vi "UnittodB.vi"   [LabVIEW 2014]
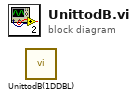
[diagram p0: block diagram]
diagram:
  n1 = call "UnittodB(1DDBL).vi"() -> ()  [unwired: 11 in, 1 out]
